vi "SolarPanel.vi"() -> ()   [LabVIEW 2013]
panel:
  out "Photocell 2-2":dbl
  out "Photocell 2-1":dbl
  out "Photocell 1-2":dbl
  out "Photocell 1-1":dbl
  in  "?":bool
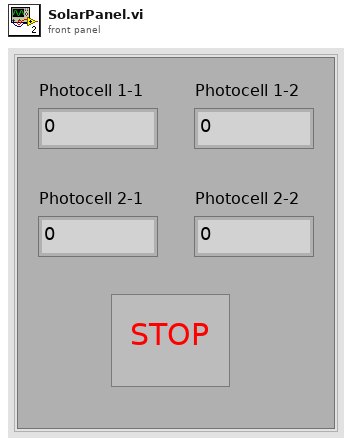
[diagram p1: front panel]
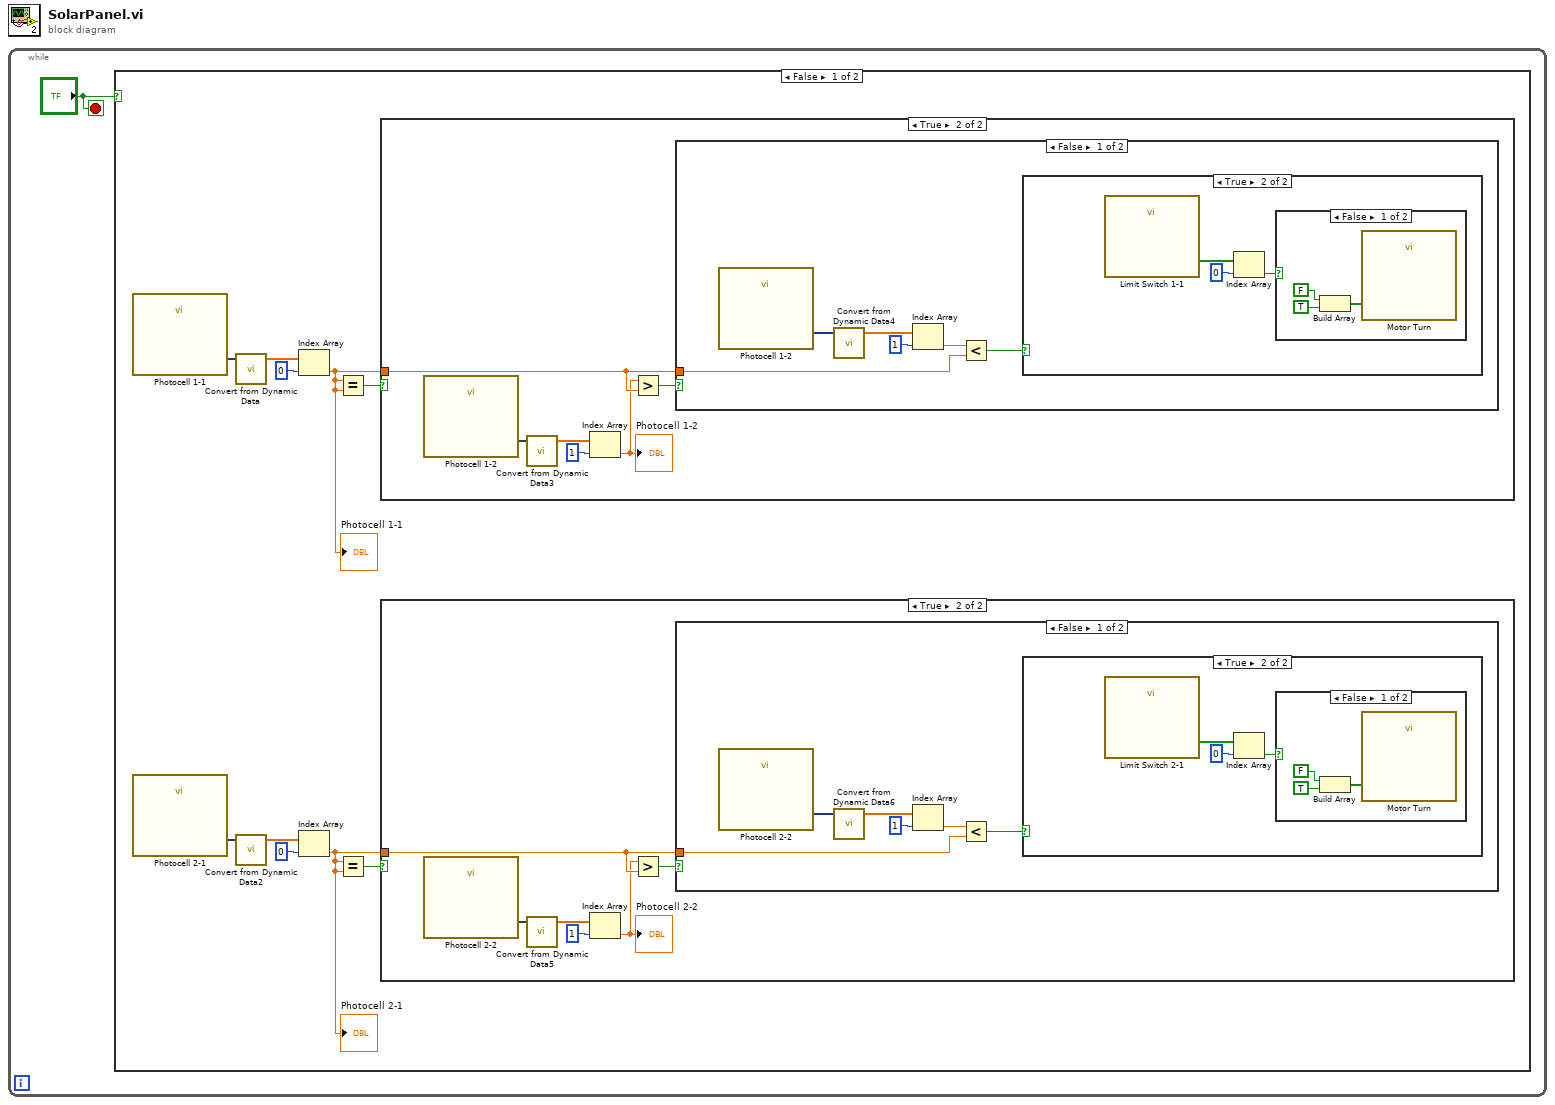
[diagram p0: block diagram]
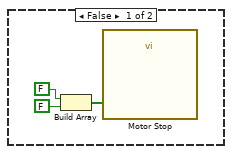
[diagram p3: hidden frame]
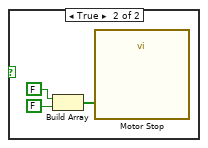
[diagram p4: hidden frame]
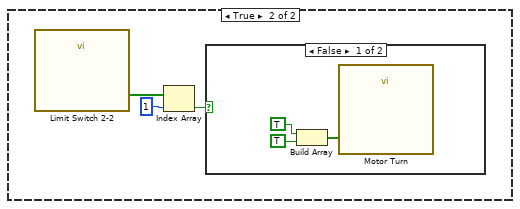
[diagram p5: hidden frame]
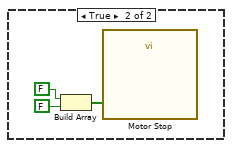
[diagram p6: hidden frame]
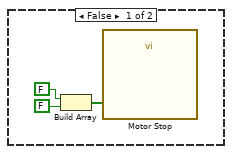
[diagram p8: hidden frame]
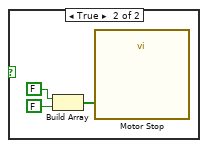
[diagram p9: hidden frame]
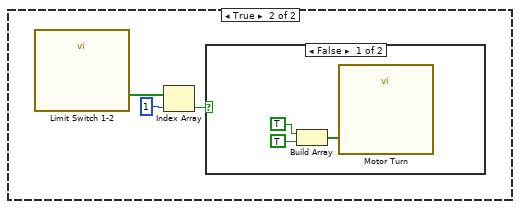
[diagram p10: hidden frame]
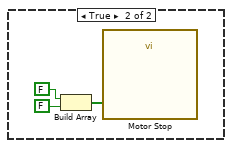
[diagram p11: hidden frame]
diagram:
  n1 = while {
    stop <- "?" stop-if-true
    n2 = case shown="False" "?" {
      frame False {
        n3 = call "Photocell 1-1"() -> ("data"=w11:dynamicdata)  [unwired: 17 in, 2 out]
        n4 = call "Photocell 2-1"() -> ("data"=w8:dynamicdata)  [unwired: 17 in, 2 out]
        n5 = call "Convert from Dynamic Data"("Dynamic Data Type"=w11) -> ("Array"=w10:dbl[])  [unwired: 3 in]
        n6 = call "Convert from Dynamic Data2"("Dynamic Data Type"=w8) -> ("Array"=w7:dbl[])  [unwired: 3 in]
        n7 = Index Array(array=w10, index=0) -> (element=w3:dbl)
        "Photocell 1-1" <- w3
        n8 = Index Array(array=w7, index=0) -> (element=w2:dbl)
        "Photocell 2-1" <- w2
        n9 = Equal?(x=w3, y=w3) -> (x = y?=w5:bool)
        n10 = Equal?(x=w2, y=w2) -> (x = y?=w4:bool)
        n11 = case shown="True" w5 {
          tunnel: w3 -> [_ w46]
          frame False {
          }
          frame True {
            n12 = call "Photocell 1-2"() -> ("data"=w50:dynamicdata)  [unwired: 17 in, 2 out]
            n13 = call "Convert from Dynamic Data3"("Dynamic Data Type"=w50) -> ("Array"=w49:dbl[])  [unwired: 3 in]
            n14 = Index Array(array=w49, index=1) -> (element=w45:dbl)
            "Photocell 1-2" <- w45
            n15 = Greater?(x=w45, y=w46) -> (0:w47:bool)
            n16 = case shown="False" w47 {
              tunnel: w46 -> [w52 _]
              frame False {
                n17 = call "Photocell 1-2"() -> ("data"=w56:dynamicdata)  [unwired: 17 in, 2 out]
                n18 = call "Convert from Dynamic Data4"("Dynamic Data Type"=w56) -> ("Array"=w55:dbl[])  [unwired: 3 in]
                n19 = Index Array(array=w55, index=1) -> (element=w53:dbl)
                n20 = Less?(x=w53, y=w52) -> (x < y?=w51:bool)
                n21 = case shown="True" w51 {
                  frame False {
                    n22 = Build Array(FALSE, FALSE) -> (w59:bool[])
                    n23 = call "Motor Stop"("data"=w59) -> ()  [unwired: 17 in, 2 out]
                  }
                  frame True {
                    n24 = call "Limit Switch 1-1"() -> ("data"=w62:bool[])  [unwired: 17 in, 2 out]
                    n25 = Index Array(array=w62, index=0) -> (element=w60:bool)
                    n26 = case shown="False" w60 {
                      frame False {
                        n27 = Build Array(FALSE, TRUE) -> (w65:bool[])
                        n28 = call "Motor Turn"("data"=w65) -> ()  [unwired: 17 in, 2 out]
                      }
                      frame True {
                        n29 = Build Array(FALSE, FALSE) -> (w68:bool[])
                        n30 = call "Motor Stop"("data"=w68) -> ()  [unwired: 17 in, 2 out]
                      }
                    }
                  }
                }
              }
              frame True {
                n31 = call "Limit Switch 1-2"() -> ("data"=w71:bool[])  [unwired: 17 in, 2 out]
                n32 = Index Array(array=w71, index=1) -> (element=w69:bool)
                n33 = case shown="False" w69 {
                  frame False {
                    n34 = Build Array(TRUE, TRUE) -> (w74:bool[])
                    n35 = call "Motor Turn"("data"=w74) -> ()  [unwired: 17 in, 2 out]
                  }
                  frame True {
                    n36 = Build Array(FALSE, FALSE) -> (w77:bool[])
                    n37 = call "Motor Stop"("data"=w77) -> ()  [unwired: 17 in, 2 out]
                  }
                }
              }
            }
          }
        }
        n38 = case shown="True" w4 {
          tunnel: w2 -> [_ w13]
          frame False {
          }
          frame True {
            n39 = call "Photocell 2-2"() -> ("data"=w17:dynamicdata)  [unwired: 17 in, 2 out]
            n40 = call "Convert from Dynamic Data5"("Dynamic Data Type"=w17) -> ("Array"=w16:dbl[])  [unwired: 3 in]
            n41 = Index Array(array=w16, index=1) -> (element=w12:dbl)
            "Photocell 2-2" <- w12
            n42 = Greater?(x=w12, y=w13) -> (0:w14:bool)
            n43 = case shown="False" w14 {
              tunnel: w13 -> [w19 _]
              frame False {
                n44 = call "Photocell 2-2"() -> ("data"=w23:dynamicdata)  [unwired: 17 in, 2 out]
                n45 = call "Convert from Dynamic Data6"("Dynamic Data Type"=w23) -> ("Array"=w22:dbl[])  [unwired: 3 in]
                n46 = Index Array(array=w22, index=1) -> (element=w20:dbl)
                n47 = Less?(x=w20, y=w19) -> (x < y?=w18:bool)
                n48 = case shown="True" w18 {
                  frame False {
                    n49 = Build Array(FALSE, FALSE) -> (w26:bool[])
                    n50 = call "Motor Stop"("data"=w26) -> ()  [unwired: 17 in, 2 out]
                  }
                  frame True {
                    n51 = call "Limit Switch 2-1"() -> ("data"=w29:bool[])  [unwired: 17 in, 2 out]
                    n52 = Index Array(array=w29, index=0) -> (element=w27:bool)
                    n53 = case shown="False" w27 {
                      frame False {
                        n54 = Build Array(FALSE, TRUE) -> (w32:bool[])
                        n55 = call "Motor Turn"("data"=w32) -> ()  [unwired: 17 in, 2 out]
                      }
                      frame True {
                        n56 = Build Array(FALSE, FALSE) -> (w35:bool[])
                        n57 = call "Motor Stop"("data"=w35) -> ()  [unwired: 17 in, 2 out]
                      }
                    }
                  }
                }
              }
              frame True {
                n58 = call "Limit Switch 2-2"() -> ("data"=w38:bool[])  [unwired: 17 in, 2 out]
                n59 = Index Array(array=w38, index=1) -> (element=w36:bool)
                n60 = case shown="False" w36 {
                  frame False {
                    n61 = Build Array(TRUE, TRUE) -> (w41:bool[])
                    n62 = call "Motor Turn"("data"=w41) -> ()  [unwired: 17 in, 2 out]
                  }
                  frame True {
                    n63 = Build Array(FALSE, FALSE) -> (w44:bool[])
                    n64 = call "Motor Stop"("data"=w44) -> ()  [unwired: 17 in, 2 out]
                  }
                }
              }
            }
          }
        }
      }
      frame True {
      }
    }
  }
